vi "test_OneSessTwoPinOneInstrOneSiteReservation_CallNiDcPowerGetConnections1PinMConnections_ReturnsTwoConnections.vi"(8 "error in":errorcluster) -> (0 "error out":errorcluster, 2 "result":string, 3 "pass":bool)   [LabVIEW 2020, in "MeasurementServerTests.lvlib"]
uses:
  MeasurementServerTests.lvlib
  Runtime/MeasurementLink Session Management V1/Session Reservation/Connection.ctl
  Runtime/MeasurementLink niDCPower/Connection with Session.ctl
  a536e905-e99b-4ce6-9f7b-add65bd26abc.vi
  03fc85e1-696b-4ece-a78b-f41470766ac0.vi
  Runtime/MeasurementLink niDCPower/Get Connections - 1Pin MConn.vi
  Runtime/MeasurementLink Session Management V1/Session Reservation/Session Reservation.lvclass
  Runtime/MeasurementLink niDCPower/MeasurementLink niDCPower.lvlib
  37c859c8-e4f6-4872-a9f8-0d1988c85ee3.vi
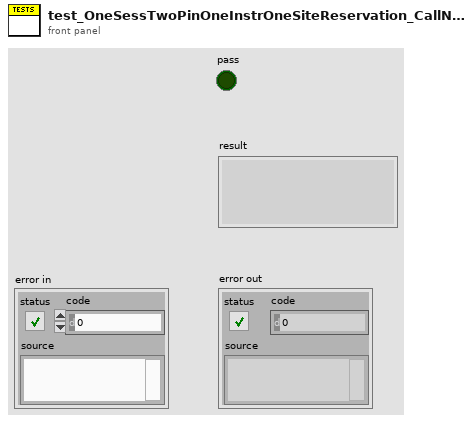
[diagram p1: front panel]
types:
  T1 = typedef "MeasurementLink Session Management V1.lvlib/Session Reservation.lvclass/Connection.ctl" = cluster{"pin or relay name":string, "site":i32, "instrument type id":string, "channel":string}
  T2 = typedef "MeasurementLink niDCPower.lvlib/Connection with Session.ctl" = cluster{"connection":T1, "session":refnum<k15>}
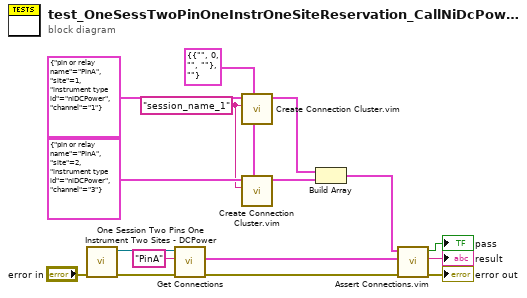
[diagram p0: block diagram]
diagram:
  w9 = T2 {"connection"={"pin or relay name"="", "site"=0, "instrument type id"="", "channel"=""}, "session"=""} ("niDCPower connection")
  w8 = "session_name_1" ("session in")
  n1 = call "One Session Two Pins One Instrument Two Sites - DCPower.vi"("error in"="error in") -> ("error out"=w4:errorcluster, "session reservation out"=w3:refnum<class "Session Reservation.lvclass">)  [unwired: 9 in]
  n2 = call-poly "Get Connections.vi"("error in"=w4, "pin or relay name"="PinA", "session reservation in"=w3) -> ("error out"=w2:errorcluster, "connections"=w16:T2[])  [unwired: 6 in, 1 out]
  n3 = call "Create Connection Cluster.vim"("connection type"=w9, "session in"=w8, "hardware independent connection in"=T1 {"pin or relay name"="PinA", "site"=1, "instrument type id"="niDCPower", "channel"="1"} ("connection")) -> ("connection out"=w7:T2)  [unwired: 8 in]
  n4 = call "Create Connection Cluster.vim"("connection type"=w9, "session in"=w8, "hardware independent connection in"=T1 {"pin or relay name"="PinA", "site"=2, "instrument type id"="niDCPower", "channel"="3"} ("connection")) -> ("connection out"=w6:T2)  [unwired: 8 in]
  n5 = Build Array(w7, w6) -> (w5:T2[])
  n6 = call "Assert Connections.vim"("error in"=w2, "actual connections"=w16, "expected connections"=w5) -> ("error out"=→"error out":errorcluster, "result"=→"result":string, "pass"=→"pass":bool)  [unwired: 6 in]
